vi "NR Configure Common.vi"(0 "RFmx Handle In":refnum<k21>, 1 "Selector String":string, 5 "Common Configuration":T1={"Center Frequency (Hz)"=3500000000.0, "Reference Level (dBm)"=0.0, "External Attenuation (dB)"=0.0, "Trigger Enabled"=TRUE, "Digital Trigger Source"="PXI_Trig0", "Trigger Delay (s)"=0.0, "Selected Ports"=""} {"Trigger Delay (s)" format="%.2p"; "External Attenuation (dB)" format="%.2f"; "Reference Level (dBm)" format="%.2f"; "Center Frequency (Hz)" format="%.6p"}, 11 "error in (no error)":errorcluster) -> (4 "RFmx Handle Out":refnum<k21>, 15 "error out":errorcluster)   [LabVIEW 2016, in "RFmxNR.lvlib"]
uses:
  RFmxNR.lvlib
  Common/SA Common Configuration.ctl
  <vilib>/RFmx/NR/mx/RFmxNR.llb/RFmxNR Configure Digital Edge Trigger.vi
  <resource>/objmgr/RFmxNR.rc
  Common/Common.lvlib
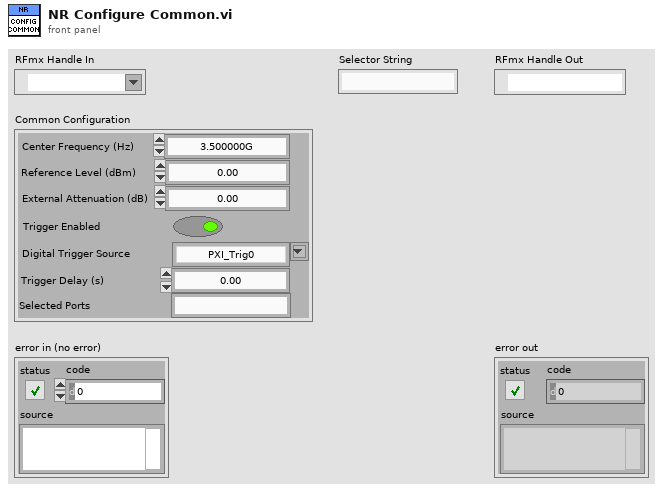
[diagram p1: front panel]
types:
  T1 = typedef "Common.lvlib/SA Common Configuration.ctl" = cluster{"Center Frequency (Hz)":dbl, "Reference Level (dBm)":dbl, "External Attenuation (dB)":dbl, "Trigger Enabled":bool, "Digital Trigger Source":string, "Trigger Delay (s)":dbl, "Selected Ports":string}
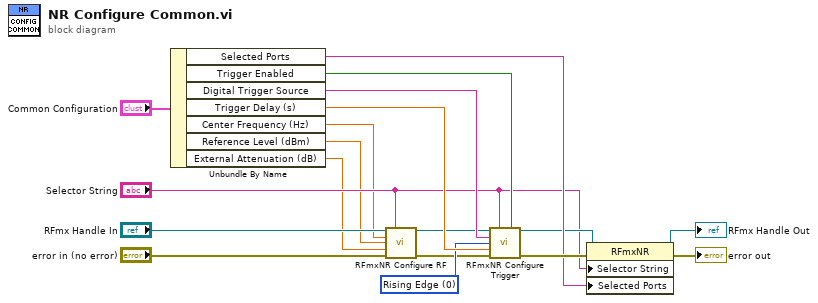
[diagram p0: block diagram]
diagram:
  w10 = 0 items=["Rising Edge", "Falling Edge"] ("Digital Edge")
  n1 = Unbundle By Name("Common Configuration") -> ("Selected Ports"=w9:string, "Trigger Enabled"=w13:bool, "Digital Trigger Source"=w14:string, "Trigger Delay (s)"=w15:dbl, "Center Frequency (Hz)"=w3:dbl, "Reference Level (dBm)"=w2:dbl, "External Attenuation (dB)"=w1:dbl)
  n2 = call <vilib>:"RFmxNR Configure RF.vi"("Instrument Handle In"="RFmx Handle In", "Selector String"="Selector String", "Center Frequency (Hz)"=w3, "Reference Level"=w2, "External Attenuation (dB)"=w1, "error in (no error)"="error in (no error)") -> ("Instrument Handle Out"=w6:refnum<k21>, "error out"=w5:errorcluster)  [unwired: 8 in]
  n3 = call-poly <vilib>:"RFmxNR Configure Trigger.vi"("Instrument Handle In"=w6, "Selector String"="Selector String", "Enable Trigger?"=w13, "Digital Edge Source"=w14, "Digital Edge"=w10, "Trigger Delay (s)"=w15, "error in (no error)"=w5) -> ("Instrument Handle Out"=w8:refnum<k21>, "error out"=w16:errorcluster)  [unwired: 7 in]
  n4 = property class="RFmxNR"(reference=w8, error in=w16, "Selector String"="Selector String", "Selected Ports"=w9) -> (reference out=→"RFmx Handle Out":refnum<k21>, error out=→"error out":errorcluster)
